vi "UiCharts_b2g2.vi"() -> ()   [LabVIEW 2011]
uses:
  Output - Cluster b2g2.ctl
  Input - Cluster b2g2.ctl
  DBSqlSelectToArray(2DArrayString).vi
panel:
  in  "Tab Control":T1(tab)
  out "protocol":string[][](table)
  out "pH-Wert":dbl(graph)
  out "Temperaturregelung":T2(graph)
  out "Füllstandsregelung":T3(graph)
  out "Druckregelung":T4(graph)
  in  "load":bool
  out "XY Graph":cluster{timestamp, dbl}[](graph)
  in  "end":timestamp=timestamp(3427221599.999 s since 1904-01-01) format="%<%X\n%x>T"
  in  "begin":timestamp=timestamp(3427135200 s since 1904-01-01) format="%<%X\n%x>T"
  in  "sensor":T5(ring)
  in  "plant":enum16{"B2G1", "B2G2"}(ring)=enum."B2G2"
  out "error out":errorcluster
  in  "stop":bool
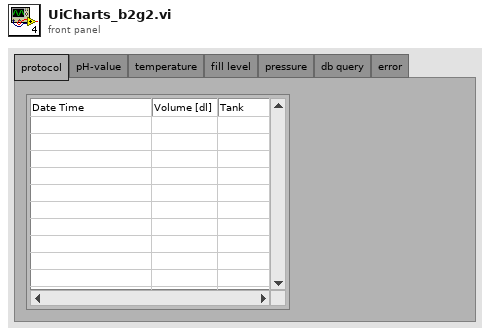
[diagram p1: front panel]
types:
  T1 = enum32{"protocol", "pH-value", "temperature", "fill level", "pressure", "db query", "error"}
  T2 = cluster{"Temp Soll [°C]":sgl, "TS-4 [°C]":dbl, dbl, dbl}
  T3 = cluster{"Füllstand Soll [l]":sgl, "FS-3 [l]":dbl, dbl}
  T4 = cluster{"Druck Soll [bar]":sgl, "DS-1 [bar]":dbl, dbl, dbl}
  T5 = enum16{"pressure", "temperature 4", "temperature 5", "pH-value", "fill level 1", "fill level 2", "fill level 3"}
  T6 = typedef "Input - Cluster b2g2.ctl" = cluster{"V-13 [%]":u8, "V-15 [%]":u8, "Log-Target":bool, "P-4":bool, "P-4 Drehzahl [%]":u8, "Temperaturregelung":bool, "Überdruckregelung":bool, "Füllstandsregulierung":bool, "V-10":bool, "Log-Host":bool, "V-14":bool, "HS-1":bool, "Füllstand  P":sgl, "Füllstand I":sgl, "Füllstand D":sgl, "Füllstand Soll [l]":sgl, "Druck  P":sgl, "Druck I":sgl, "Druck D":sgl, "Druck Soll [bar]":sgl, "Temp Soll [°C]":sgl, "Dosierung":bool, "Dosiermenge [l]":sgl, "Dosiergeschw. [l/min]":sgl, "Tank":bool, "Hysterese [°C]":sgl, "MR Füllstandsüberwachung":bool, "Tank Füllstandsüberwachung":bool, "Log Target [ms]":u32, "Log Host [s]":u32, "Zirkulation EIN [min]":u8, "Zirkulation AUS [min]":u8, "Zirkulation":bool, "V-33":bool, "V-34":bool, "V-35":bool, "T1 Max Füllstand":bool, "T1 Min Füllstand":bool, "FS-1 [l]":sgl, "P-9":bool}
  T7 = typedef "Output - Cluster b2g2.ctl" = cluster{"DFS-1 [dl]":u64, "FS-3 [l]":dbl, "DFS-1 [l/min]":dbl, "DS-1 [bar]":dbl, "V-10 ZU":bool, "V-14 ZU":bool, "FS-1 [l]":dbl, "FS-2 [l]":dbl, "TS-4 [°C]":dbl, "HS-1":bool, "V-13 [%]":u8, "V-15 [%]":u8, "P-4 [%]":u8, "Dosierung":bool, "MR Max Füllstand":bool, "MR Min Füllstand":bool, "Dosiermenge [l]":sgl, "V-14 AUF":bool, "V-10 AUF":bool, "T-1 Max Füllstand":bool, "T-1 Min Füllstand":bool, "T-2 Max Füllstand":bool, "T-2 Min Füllstand":bool, "pHS-1 [pH]":dbl, "P-4 RUN":bool, "V-33 AUF":bool, "V-33 ZU":bool, "V-34 AUF":bool, "V-34 ZU":bool, "P-4 ERR":bool, "TS-5 [°C]":dbl, "V-35 AUF":bool, "V-35 ZU":bool, "P-9 RUN":bool}
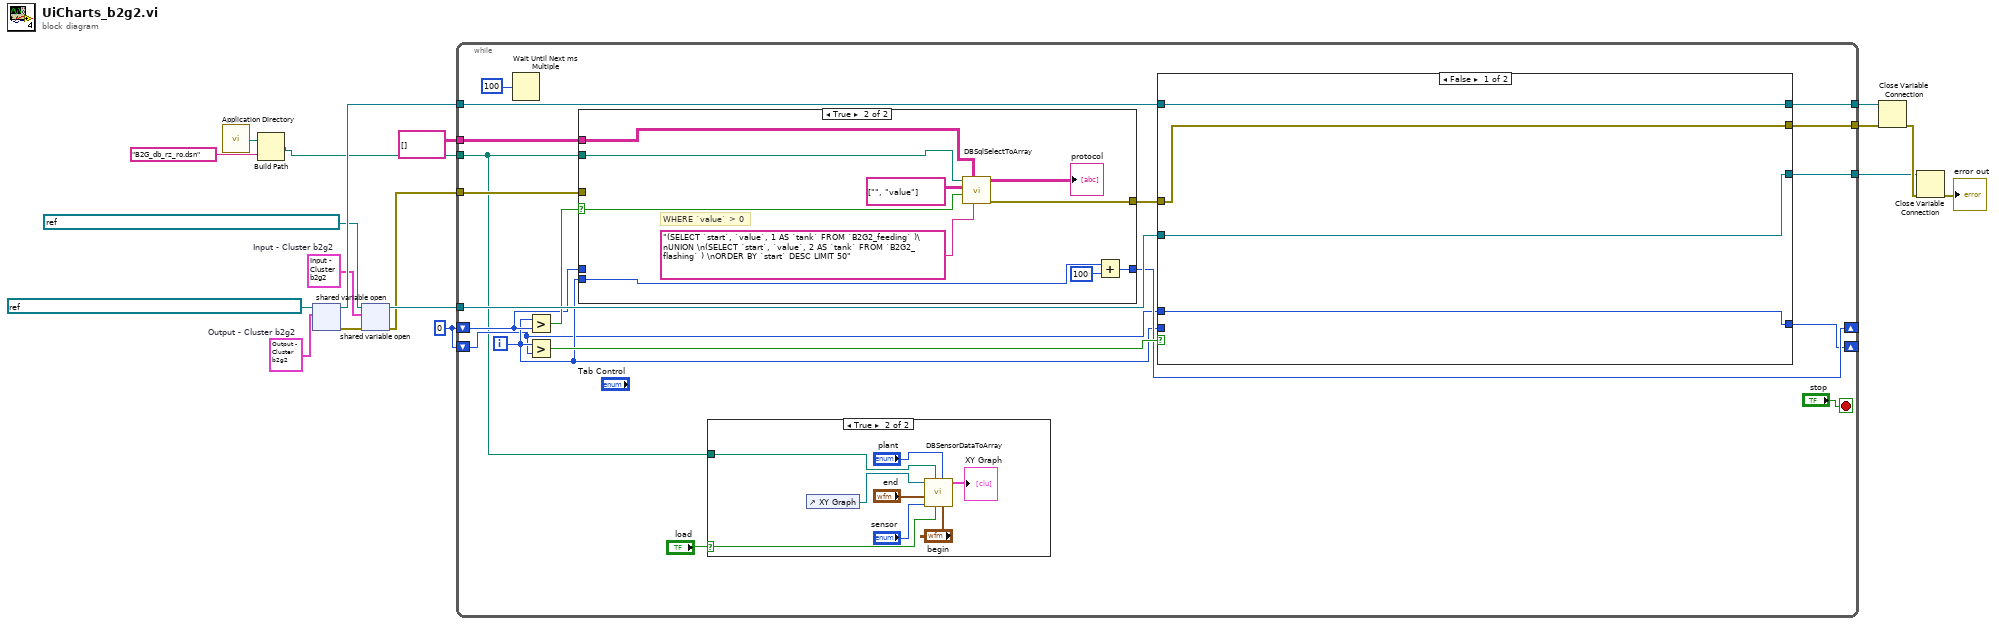
[diagram p0: block diagram]
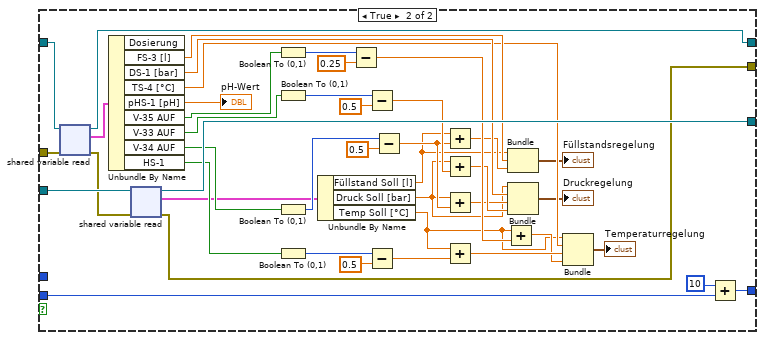
[diagram p4: hidden frame]
diagram:
  w14 = T6 {"V-13 [%]"=0, "V-15 [%]"=0, "Log-Target"=FALSE, "P-4"=FALSE, "P-4 Drehzahl [%]"=0, "Temperaturregelung"=FALSE, "Überdruckregelung"=FALSE, "Füllstandsregulierung"=FALSE, "V-10"=FALSE, "Log-Host"=FALSE, "V-14"=FALSE, "HS-1"=FALSE, "Füllstand  P"=0.0, "Füllstand I"=0.0, "Füllstand D"=0.0, "Füllstand Soll [l]"=0.0, "Druck  P"=0.0, "Druck I"=0.0, "Druck D"=0.0, "Druck Soll [bar]"=0.0, "Temp Soll [°C]"=0.0, "Dosierung"=FALSE, "Dosiermenge [l]"=0.0, "Dosiergeschw. [l/min]"=0.0, "Tank"=FALSE, "Hysterese [°C]"=0.0, "MR Füllstandsüberwachung"=FALSE, "Tank Füllstandsüberwachung"=FALSE, "Log Target [ms]"=0, "Log Host [s]"=0, "Zirkulation EIN [min]"=0, "Zirkulation AUS [min]"=0, "Zirkulation"=FALSE, "V-33"=FALSE, "V-34"=FALSE, "V-35"=FALSE, "T1 Max Füllstand"=FALSE, "T1 Min Füllstand"=FALSE, "FS-1 [l]"=0.0, "P-9"=FALSE}  # Input - Cluster b2g2
  w17 = T7 {"DFS-1 [dl]"=0, "FS-3 [l]"=0.0, "DFS-1 [l/min]"=0.0, "DS-1 [bar]"=0.0, "V-10 ZU"=FALSE, "V-14 ZU"=FALSE, "FS-1 [l]"=0.0, "FS-2 [l]"=0.0, "TS-4 [°C]"=0.0, "HS-1"=FALSE, "V-13 [%]"=0, "V-15 [%]"=0, "P-4 [%]"=0, "Dosierung"=FALSE, "MR Max Füllstand"=FALSE, "MR Min Füllstand"=FALSE, "Dosiermenge [l]"=0.0, "V-14 AUF"=FALSE, "V-10 AUF"=FALSE, "T-1 Max Füllstand"=FALSE, "T-1 Min Füllstand"=FALSE, "T-2 Max Füllstand"=FALSE, "T-2 Min Füllstand"=FALSE, "pHS-1 [pH]"=0.0, "P-4 RUN"=FALSE, "V-33 AUF"=FALSE, "V-33 ZU"=FALSE, "V-34 AUF"=FALSE, "V-34 ZU"=FALSE, "P-4 ERR"=FALSE, "TS-5 [°C]"=0.0, "V-35 AUF"=FALSE, "V-35 ZU"=FALSE, "P-9 RUN"=FALSE}  # Output - Cluster b2g2
  w6 = i64 0
  n1 = call <vilib>:"Application Directory.vi"() -> ("Application Directory"=w3:path)
  n2 = Build Path(base path=w3, name or relative path="B2G_db_rz_ro.dsn" ("Name of ini file 2")) -> (appended path=w1:path)
  n3 = shared-variable-open(refnum<k21> "ni.var.psp://10.27.40.25/variables - b2g2/data - network b2g2" ("Output Var"), w17) -> (w16:refnum<k21>, w11:errorcluster)  [unwired: 2 in]
  n4 = shared-variable-open(refnum<k21> "ni.var.psp://10.27.40.25/variables - b2g2/input - network b2g2" ("Input Var"), w11, w14) -> (w12:refnum<k21>, w5:errorcluster)  [unwired: 1 in]
  n5 = while {
    tunnel: w16 -> [w37]
    tunnel: [w36] -> w15
    tunnel: w12 -> [w35]
    tunnel: [w34] -> w9
    tunnel: string[][] [] ("data") -> [w33]
    shift-right: [w29] -> _
    shift-left: w6 -> [w30]
    shift-right: [w28] -> _
    shift-left: w6 -> [w25]
    tunnel: w5 -> [w21]
    tunnel: [w20] -> w4
    tunnel: w1 -> [w19]
    i -> [w26]
    stop <- "stop" stop-if-true
    n6 = Wait Until Next ms Multiple(millisecond multiple=100) -> ()  [unwired: 1 out]
    n7 = Greater?(x=w26, y=w30) -> (0:w32:bool)
    n8 = Greater?(x=w26, y=w25) -> (0:w31:bool)
    n9 = case shown="True" w32 {
      selector: w32 -> [_ w50]
      tunnel: [w47 w56] -> w29
      tunnel: w30 -> [w47 _]
      tunnel: w26 -> [_ w57]
      tunnel: w33 -> [_ w53]
      tunnel: [w46 w52] -> w23
      tunnel: w21 -> [w46 _]
      tunnel: w19 -> [_ w48]
      frame False {
      }
      frame True {
        # "WHERE `value` > 0"
        n10 = call-poly "DBSqlSelectToArray.vi"("String"="(SELECT `start`, `value`, 1 AS `tank` FROM `B2G2_feeding` )\nUNION \n(SELECT `start`, `value`, 2 AS `tank` FROM `B2G2_flashing` ) \nORDER BY `start` DESC LIMIT 50" ("SQL query"), "shift reg in"=w53, "enable"=w50, "format"=string[][] [["", "value"]] ("columns"), "connection information"=w48) -> ("error out"=w52:errorcluster, "shift reg out"=→"protocol":string[][])  [unwired: 5 in]
        n11 = Add(x=w57, y=i64 100) -> (x+y=w56:i64)
      }
    }
    n12 = case shown="True" "load" {
      selector: "load" -> [_ w39]
      tunnel: w19 -> [_ w38]
      frame False {
      }
      frame True {
        n13 = control-ref of="XY Graph"() -> (w41:refnum<vi>)
        n14 = call "DBSensorDataToArray.vi"("begin"="begin", "plant"="plant", "load"=w39, "appended path"=w38, "sensor"="sensor", "end"="end", "XYGraph in"=w41) -> ("shift reg out"=→"XY Graph":cluster{timestamp, dbl}[])  [unwired: 3 in, 1 out]
      }
    }
    n15 = case shown="False" w31 {
      tunnel: w37 -> [w60 w104]
      tunnel: [w60 w103] -> w36
      tunnel: w35 -> [w59 w102]
      tunnel: [w59 w101] -> w34
      tunnel: [w61 w65] -> w28
      tunnel: w26 -> [_ w64]
      tunnel: w25 -> [w61 _]
      tunnel: w23 -> [w58 w63]
      tunnel: [w58 w62] -> w20
      frame False {
      }
      frame True {
        n16 = shared-variable-read(w104, w63) -> (w103:refnum<k21>, w71:errorcluster, w100:T7)  [unwired: 1 out]
        n17 = Unbundle By Name(w100) -> ("FS-3 [l]"=w99:dbl, "DS-1 [bar]"=w98:dbl, "TS-4 [°C]"=w97:dbl, "pHS-1 [pH]"=→"pH-Wert":dbl, "V-35 AUF"=w93:bool, "V-33 AUF"=w95:bool, "V-34 AUF"=w94:bool, "HS-1"=w92:bool)  [unwired: 1 out]
        n18 = shared-variable-read(w102, w71) -> (w101:refnum<k21>, w62:errorcluster, w70:T6)  [unwired: 1 out]
        n19 = Boolean To (0,1)(Boolean=w93) -> (0, 1=w85:i16)
        n20 = Boolean To (0,1)(Boolean=w95) -> (0, 1=w76:i16)
        n21 = Boolean To (0,1)(Boolean=w94) -> (0, 1=w75:i16)
        n22 = Boolean To (0,1)(Boolean=w92) -> (0, 1=w88:i16)
        n23 = Unbundle By Name(w70) -> ("Füllstand Soll [l]"=w69:sgl, "Druck Soll [bar]"=w67:sgl, "Temp Soll [°C]"=w68:sgl)
        n24 = Subtract(x=w85, y=0.25) -> (x-y=w87:dbl)
        n25 = Subtract(x=w76, y=0.5) -> (x-y=w83:dbl)
        n26 = Subtract(x=w88, y=0.5) -> (x-y=w91:dbl)
        n27 = Subtract(x=w75, y=0.5) -> (x-y=w77:dbl)
        n28 = Add(x=w69, y=w77) -> (x+y=w78:dbl)
        n29 = Add(x=w67, y=w83) -> (x+y=w81:dbl)
        n30 = Add(x=w67, y=w77) -> (x+y=w79:dbl)
        n31 = Add(x=w68, y=w91) -> (x+y=w90:dbl)
        n32 = Add(x=w68, y=w87) -> (x+y=w84:dbl)
        n33 = Bundle("Füllstand Soll [l]"=w69, "FS-3 [l]"=w99, w78) -> (→"Füllstandsregelung":T3)  [unwired: 1 in]
        n34 = Bundle("Druck Soll [bar]"=w67, "DS-1 [bar]"=w98, w79, w81) -> (→"Druckregelung":T4)  [unwired: 1 in]
        n35 = Bundle("Temp Soll [°C]"=w68, "TS-4 [°C]"=w97, w90, w84) -> (→"Temperaturregelung":T2)  [unwired: 1 in]
        n36 = Add(x=10, y=w64) -> (x+y=w65:i32)
      }
    }
  }
  n37 = Close Variable Connection(8:w4, 11:w15) -> (0:w10:errorcluster)
  n38 = Close Variable Connection(8:w10, 11:w9) -> (0:→"error out":errorcluster)
